vi "NiXnet ReadState.vi"(6 "contextId":T1, 8 "error in":errorcluster, 9 "timeout (ms)":i32=-1, 10 "Request Data":T4, 11 "gRPC ID":T1) -> (0 "error out":errorcluster, 2 "Response Data":T2, 3 "gRPC ID out":T1)   [LabVIEW 2025, in "xnet-grpc_client.lvlib"]
uses:
  xnet-grpc_client.lvlib
  <vilib>/gRPC/LabVIEW gRPC Library/Shared/grpcId.ctl
  RPC Messages/nixnet_grpc_ReadStateRequest.ctl
  RPC Messages/nixnet_grpc_ReadStateRequest_state_id_enum/nixnet_grpc_ReadStateRequest_state_id_enum.lvclass
  RPC Messages/nidevice_grpc_Session.ctl
  RPC Messages/nixnet_grpc_ReadStateResponse.ctl
  RPC Messages/nixnet_grpc_ReadStateValue_value/nixnet_grpc_ReadStateValue_value.lvclass
  RPC Messages/nixnet_grpc_ReadStateValue.ctl
  RPC Messages/nixnet_grpc_ReadStateResponse_Flat.ctl
  RPC Messages/nixnet_grpc_ReadStateValue_Flat.ctl
  RPC Messages/nixnet_grpc_CanCommResponse_Flat.ctl
  RPC Messages/nixnet_grpc_CanCommState.ctl
  RPC Messages/nixnet_grpc_CanLastErr.ctl
  RPC Messages/nixnet_grpc_FlexRayCommResponse_Flat.ctl
  RPC Messages/nixnet_grpc_FlexRayPocState.ctl
  RPC Messages/nixnet_grpc_FlexRayStats_Flat.ctl
  RPC Messages/nixnet_grpc_LinCommResponse_Flat.ctl
  RPC Messages/nixnet_grpc_LinCommState.ctl
  RPC Messages/nixnet_grpc_SessionInfoResponse_Flat.ctl
  RPC Messages/nixnet_grpc_SessionInfoState.ctl
  RPC Messages/nixnet_grpc_J1939CommState_Flat.ctl
  RPC Messages/nixnet_grpc_TimeLocalNetwork_Flat.ctl
  RPC Messages/nixnet_grpc_ReadStateRequest_state_id_enum/nixnet_grpc_ReadStateRequest_state_id_enum.lvclass/nixnet_grpc_ReadStateRequest_state_id_enum.ctl
  RPC Messages/nixnet_grpc_ReadStateValue_value/nixnet_grpc_ReadStateValue_value.lvclass/nixnet_grpc_ReadStateValue_value.ctl
  14035477-4c25-4107-8ed5-d0c4ef420ce5.vi
  RPC Messages/RichToFlatnidevice_grpc_Session.vi
  RPC Messages/nixnet_grpc_ReadStateRequest_state_id_enum/GetActiveFieldIndex.vi
  RPC Messages/nixnet_grpc_ReadStateRequest_state_id_enum/Getstate_id.vi
  RPC Messages/nixnet_grpc_ReadStateRequest_state_id_enum/Getstate_id_raw.vi
  <vilib>/gRPC/LabVIEW gRPC Library/Shared/TranslateGrpcError.vi
  <vilib>/gRPC/LabVIEW gRPC Library/Shared/Wait On Occurrence Wrapper.vi
  RPC Messages/FlatToRichnixnet_grpc_ReadStateValue.vi
  <vilib>/gRPC/LabVIEW gRPC Library/Shared/Wait On Occurence.vi
  RPC Messages/nixnet_grpc_ReadStateValue_value/Settime_current.vi
  RPC Messages/nixnet_grpc_ReadStateValue_value/Settime_communicating.vi
  RPC Messages/nixnet_grpc_ReadStateValue_value/Settime_start.vi
  RPC Messages/nixnet_grpc_ReadStateValue_value/Setcan_comm.vi
  RPC Messages/FlatToRichnixnet_grpc_CanCommResponse.vi
  RPC Messages/nixnet_grpc_ReadStateValue_value/Setflex_ray_comm.vi
  RPC Messages/FlatToRichnixnet_grpc_FlexRayCommResponse.vi
  RPC Messages/nixnet_grpc_ReadStateValue_value/Setflex_ray_stats.vi
  RPC Messages/FlatToRichnixnet_grpc_FlexRayStats.vi
  RPC Messages/nixnet_grpc_ReadStateValue_value/Setlin_comm.vi
  RPC Messages/FlatToRichnixnet_grpc_LinCommResponse.vi
  RPC Messages/nixnet_grpc_ReadStateValue_value/Setsession_info.vi
  RPC Messages/FlatToRichnixnet_grpc_SessionInfoResponse.vi
  RPC Messages/nixnet_grpc_ReadStateValue_value/Setj1939_comm_state.vi
  RPC Messages/FlatToRichnixnet_grpc_J1939CommState.vi
  RPC Messages/nixnet_grpc_ReadStateValue_value/Settime_current2.vi
  RPC Messages/FlatToRichnixnet_grpc_TimeLocalNetwork.vi
  RPC Messages/nixnet_grpc_ReadStateValue_value/Settime_communicating2.vi
  RPC Messages/nixnet_grpc_ReadStateValue_value/Settime_start2.vi
  <vilib>/gRPC/LabVIEW gRPC Library/Server API/Server/Get Server DLL Path.vi
  <vilib>/Utility/error.llb/Error Cluster From Error Code.vi
  <vilib>/Utility/config.llb/Open Config Data.vi
  <vilib>/Utility/config.llb/Write Key.vi
  <vilib>/Utility/config.llb/Write Key (Boolean).vi
  <vilib>/Utility/config.llb/Not A Config Data Refnum.vi
  <vilib>/Utility/config.llb/Read Key.vi
  <vilib>/Utility/config.llb/Read Key (Boolean).vi
  <vilib>/Utility/config.llb/Close Config Data.vi
  RPC Messages/nixnet_grpc_ReadStateValue_value/GetActiveFieldName.vi
  <vilib>/gRPC/LabVIEW gRPC Library/grpc-lvsupport-release.lvlib
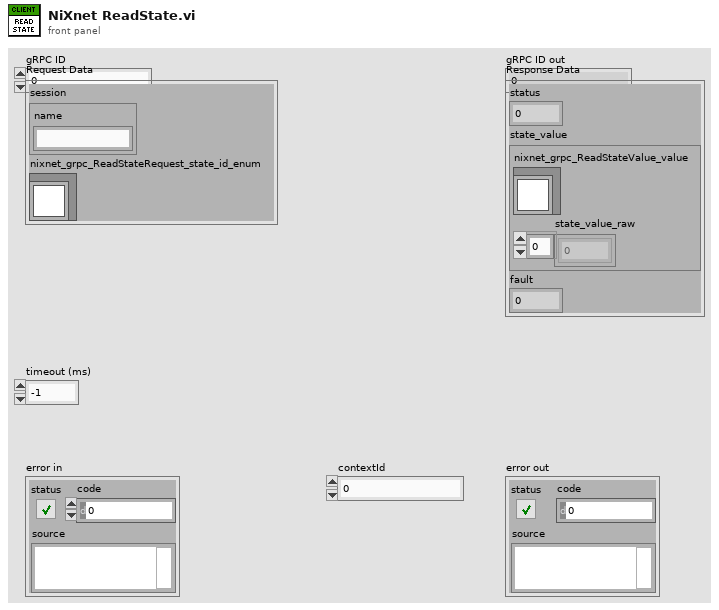
[diagram p1: front panel]
types:
  T1 = typedef "grpc-lvsupport-release.lvlib/grpcId.ctl" = u64
  T2 = typedef "xnet-grpc_client.lvlib/nixnet_grpc_ReadStateResponse.ctl" = cluster{"status":i32, "state_value":T3, "fault":i32}
  T3 = typedef "xnet-grpc_client.lvlib/nixnet_grpc_ReadStateValue.ctl" = cluster{"nixnet_grpc_ReadStateValue_value":refnum<class "nixnet_grpc_ReadStateValue_value.lvclass">, "state_value_raw":u8[]}
  T4 = typedef "xnet-grpc_client.lvlib/nixnet_grpc_ReadStateRequest.ctl" = cluster{"session":T5, "nixnet_grpc_ReadStateRequest_state_id_enum":refnum<class "nixnet_grpc_ReadStateRequest_state_id_enum.lvclass">}
  T5 = typedef "xnet-grpc_client.lvlib/nidevice_grpc_Session.ctl" = cluster{"name":string}
  T6 = typedef "xnet-grpc_client.lvlib/nixnet_grpc_ReadStateResponse_Flat.ctl" = cluster{"status":i32, "state_value":T7, "fault":i32}
  T7 = typedef "xnet-grpc_client.lvlib/nixnet_grpc_ReadStateValue_Flat.ctl" = cluster{"nixnet_grpc_ReadStateValue_value_selected_index":i32, "time_current":u64, "time_communicating":u64, "time_start":u64, "can_comm":T8, "flex_ray_comm":T11, "flex_ray_stats":T13, "lin_comm":T14, "session_info":T16, "j1939_comm_state":T18, "time_current2":T19, "time_communicating2":T19, "time_start2":T19, "state_value_raw":u8[]}
  T8 = typedef "xnet-grpc_client.lvlib/nixnet_grpc_CanCommResponse_Flat.ctl" = cluster{"comm_state":T9, "comm_state_raw":u32, "transceiver_error":u32, "sleep":u32, "last_error":T10, "last_error_raw":u32, "transmit_error_counter":u32, "receive_error_counter":u32}
  T9 = typedef "xnet-grpc_client.lvlib/nixnet_grpc_CanCommState.ctl" = enum32{"CAN_COMM_STATE_ERROR_ACTIVE", "CAN_COMM_STATE_ERROR_PASSIVE", "CAN_COMM_STATE_BUS_OFF", "CAN_COMM_STATE_INIT"}
  T10 = typedef "xnet-grpc_client.lvlib/nixnet_grpc_CanLastErr.ctl" = enum32{"CAN_LAST_ERR_NONE", "CAN_LAST_ERR_STUFF", "CAN_LAST_ERR_FORM", "CAN_LAST_ERR_ACK", "CAN_LAST_ERR_BIT_1", "CAN_LAST_ERR_BIT_0", "CAN_LAST_ERR_CRC"}
  T11 = typedef "xnet-grpc_client.lvlib/nixnet_grpc_FlexRayCommResponse_Flat.ctl" = cluster{"poc_state":T12, "poc_state_raw":u32, "clock_correction_failed":u32, "passive_to_active_count":u32, "channel_a_sleep":u32, "channel_b_sleep":u32}
  T12 = typedef "xnet-grpc_client.lvlib/nixnet_grpc_FlexRayPocState.ctl" = enum32{"FLEX_RAY_POC_STATE_DEFAULT_CONFIG", "FLEX_RAY_POC_STATE_READY", "FLEX_RAY_POC_STATE_NORMAL_ACTIVE", "FLEX_RAY_POC_STATE_NORMAL_PASSIVE", "FLEX_RAY_POC_STATE_HALT", "FLEX_RAY_POC_STATE_MONITOR", "FLEX_RAY_POC_STATE_CONFIG"}
  T13 = typedef "xnet-grpc_client.lvlib/nixnet_grpc_FlexRayStats_Flat.ctl" = cluster{"num_syntax_error_ch_a":u32, "num_syntax_error_ch_b":u32, "num_content_error_ch_a":u32, "num_content_error_ch_b":u32, "num_slot_boundary_violation_ch_a":u32, "num_slot_boundary_violation_ch_b":u32}
  T14 = typedef "xnet-grpc_client.lvlib/nixnet_grpc_LinCommResponse_Flat.ctl" = cluster{"sleep":u32, "comm_state":T15, "comm_state_raw":u32, "last_error":u32, "last_error_received":u32, "last_error_expected":u32, "last_error_id":u32, "transceiver_ready":u32, "schedule_index":u32}
  T15 = typedef "xnet-grpc_client.lvlib/nixnet_grpc_LinCommState.ctl" = enum32{"LIN_COMM_STATE_IDLE", "LIN_COMM_STATE_ACTIVE", "LIN_COMM_STATE_INACTIVE"}
  T16 = typedef "xnet-grpc_client.lvlib/nixnet_grpc_SessionInfoResponse_Flat.ctl" = cluster{"info":T17, "info_raw":u32}
  T17 = typedef "xnet-grpc_client.lvlib/nixnet_grpc_SessionInfoState.ctl" = enum32{"SESSION_INFO_STATE_STOPPED", "SESSION_INFO_STATE_STARTED", "SESSION_INFO_STATE_MIX"}
  T18 = typedef "xnet-grpc_client.lvlib/nixnet_grpc_J1939CommState_Flat.ctl" = cluster{"pgn":u32, "source_address":u32, "destination_address":u32, "transmit_error":u32, "receive_error":u32}
  T19 = typedef "xnet-grpc_client.lvlib/nixnet_grpc_TimeLocalNetwork_Flat.ctl" = cluster{"local_time":u64, "network_time":u64, "flags":u32}
  T20 = typedef "xnet-grpc_client.lvlib/nixnet_grpc_ReadStateRequest_Flat.ctl" = cluster{"session":T21, "nixnet_grpc_ReadStateRequest_state_id_enum_selected_index":i32, "state_id":T22, "state_id_raw":u32}
  T21 = typedef "xnet-grpc_client.lvlib/nidevice_grpc_Session_Flat.ctl" = cluster{"name":string}
  T22 = typedef "xnet-grpc_client.lvlib/nixnet_grpc_ReadState.ctl" = enum32{"READ_STATE_UNSPECIFIED", "READ_STATE_TIME_CURRENT", "READ_STATE_TIME_COMMUNICATING", "READ_STATE_TIME_START", "READ_STATE_SESSION_INFO", "READ_STATE_TIME_CURRENT_2", "READ_STATE_TIME_COMMUNICATING_2", "READ_STATE_TIME_START_2", "READ_STATE_CAN_COMM", "READ_STATE_FLEX_RAY_COMM", "READ_STATE_FLEX_RAY_STATS", "READ_STATE_LIN_COMM", "READ_STATE_J1939_COMM"}
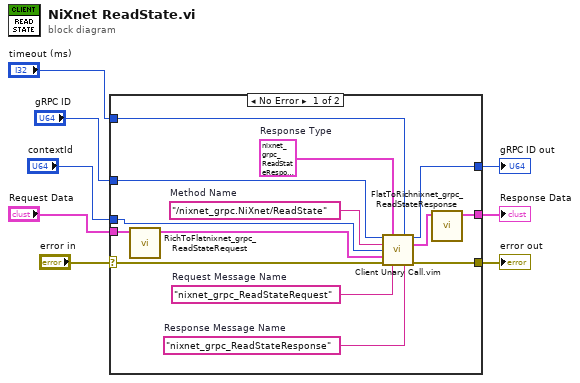
[diagram p0: block diagram]
diagram:
  n1 = case shown="No Error" "error in" {
    selector: "error in" -> [w18 w23]
    tunnel: [w17 w23] -> w7
    tunnel: "gRPC ID" -> [w16 w24]
    tunnel: [w15 w24] -> w5
    tunnel: "Request Data" -> [w12 _]
    tunnel: [w9 _] -> w3
    tunnel: "timeout (ms)" -> [w14 _]
    tunnel: "contextId" -> [w13 _]
    frame No Error {
      w19 = "nixnet_grpc_ReadStateResponse"  # Response Message Name
      w20 = "nixnet_grpc_ReadStateRequest"  # Request Message Name
      w21 = T6 {"status"=0, "state_value"={"nixnet_grpc_ReadStateValue_value_selected_index"=0, "time_current"=0, "time_communicating"=0, "time_start"=0, "can_comm"={"comm_state"=enum."CAN_COMM_STATE_ERROR_ACTIVE", "comm_state_raw"=0, "transceiver_error"=0, "sleep"=0, "last_error"=enum."CAN_LAST_ERR_NONE", "last_error_raw"=0, "transmit_error_counter"=0, "receive_error_counter"=0}, "flex_ray_comm"={"poc_state"=enum."FLEX_RAY_POC_STATE_DEFAULT_CONFIG", "poc_state_raw"=0, "clock_correction_failed"=0, "passive_to_active_count"=0, "channel_a_sleep"=0, "channel_b_sleep"=0}, "flex_ray_stats"={"num_syntax_error_ch_a"=0, "num_syntax_error_ch_b"=0, "num_content_error_ch_a"=0, "num_content_error_ch_b"=0, "num_slot_boundary_violation_ch_a"=0, "num_slot_boundary_violation_ch_b"=0}, "lin_comm"={"sleep"=0, "comm_state"=enum."LIN_COMM_STATE_IDLE", "comm_state_raw"=0, "last_error"=0, "last_error_received"=0, "last_error_expected"=0, "last_error_id"=0, "transceiver_ready"=0, "schedule_index"=0}, "session_info"={"info"=enum."SESSION_INFO_STATE_STOPPED", "info_raw"=0}, "j1939_comm_state"={"pgn"=0, "source_address"=0, "destination_address"=0, "transmit_error"=0, "receive_error"=0}, "time_current2"={"local_time"=0, "network_time"=0, "flags"=0}, "time_communicating2"={"local_time"=0, "network_time"=0, "flags"=0}, "time_start2"={"local_time"=0, "network_time"=0, "flags"=0}, "state_value_raw"=[]}, "fault"=0}  # Response Type
      w22 = "/nixnet_grpc.NiXnet/ReadState"  # Method Name
      n2 = call "RichToFlatnixnet_grpc_ReadStateRequest.vi"("InputCluster"=w12) -> ("OutputCluster"=w11:T20)  [unwired: 10 in]
      n3 = call "Client Unary Call.vim"("ClientID in"=w16, "Response Type"=w21, "timeout (ms)"=w14, "Method Name"=w22, "contextId"=w13, "Request Data"=w11, "error in"=w18, "Request Message Name"=w20, "Response Message Name"=w19) -> ("ClientID out"=w15:u64, "Response Data"=w10:T6, "error out"=w17:errorcluster)  [unwired: 4 in]
      n4 = call "FlatToRichnixnet_grpc_ReadStateResponse.vi"("InputCluster"=w10) -> ("OutputCluster"=w9:T2)  [unwired: 10 in]
    }
    frame Error {
    }
  }
  "error out" <- w7
  "gRPC ID out" <- w5
  "Response Data" <- w3
